vi "Deserialize.vi"(8 "error in (no error)":errorcluster, 10 "Serialized Message":string, 11 "Cache Manager DVR":refnum<class "Cache Manager.lvclass">) -> (0 "error out":errorcluster, 3 "Serialize out":refnum<class "Serializable Msg.lvclass">, 4 "priority":i32)   [LabVIEW 2020, in "Serializer.lvlib" / "Serializable Message.lvlib" / "Serializable Msg.lvclass"]
uses:
  Serializable Msg.lvclass
  Cache Manager/Cache Manager.lvclass
  Cache Manager/Cache Manager.lvclass/Cache Manager.ctl
  <vilib>/Utility/LVClass/Get LV Class Default Value By Name.vi
  Serializable Msg.lvclass/Serializable Msg.ctl
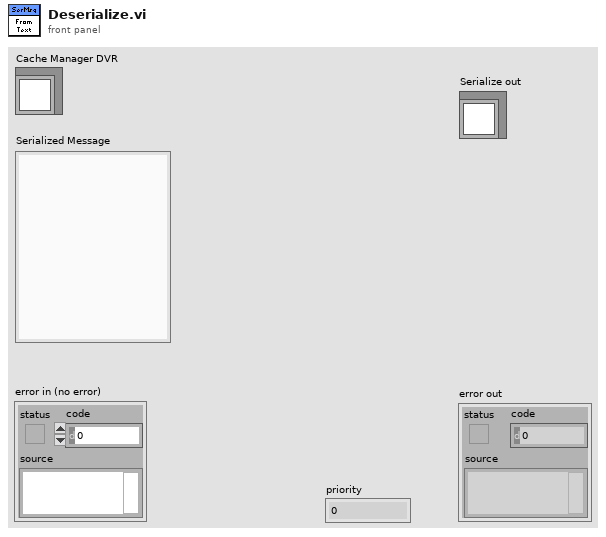
[diagram p1: front panel]
types:
  T1 = cluster{"Class name":string, "Priority":i32, "Data":string}
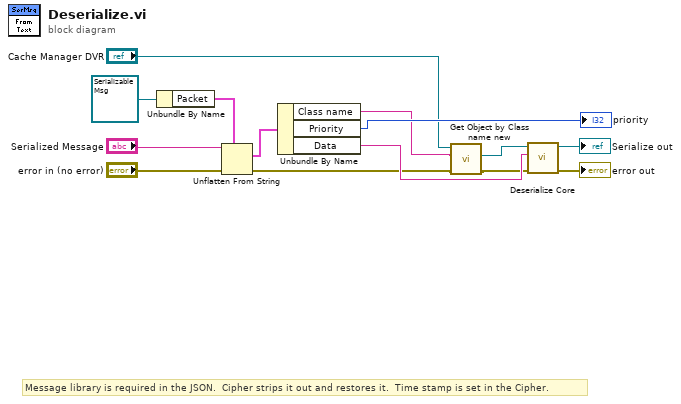
[diagram p0: block diagram]
diagram:
  # "Message library is required in the JSON.  Cipher strips it out and restores it.  Time stamp is set in the Cipher."
  n1 = Unbundle By Name(refnum<class "Serializable Msg.lvclass"> refnum ("Serialize in")) -> ("Packet"=w10:T1)
  n2 = Unflatten From String(type=w10, binary string="Serialized Message", error in (no error)="error in (no error)") -> (value=w9:T1, error out=w3:errorcluster)  [unwired: 2 in, 1 out]
  n3 = Unbundle By Name(w9) -> ("Class name"=w4:string, "Priority"=→"priority":i32, "Data"=w7:string)
  n4 = call "Get Object by Class name new.vi"("error in (no error)"=w3, "Class Name"=w4, "Cache Manager DVR in"="Cache Manager DVR") -> ("error out"=w2:errorcluster, "Serializable Message"=w1:refnum<class "Serializable Msg.lvclass">)  [unwired: 6 in, 1 out]
  n5 = call-dynamic "Deserialize Core.vi"("error in (no error)"=w2, "Serialized Attributes"=w7, "Serialize in"=w1) -> ("error out"=→"error out":errorcluster, "Serialize out"=→"Serialize out":refnum<class "Serializable Msg.lvclass">)  [unwired: 7 in]
